vi "Transistor_Test.vi"() -> ()   [LabVIEW 2020]
panel:
  in  "?":T1(tab)
  in  "?":bool=TRUE
  out "Output Characteristics":cluster{dbl[], dbl[]}[](graph)
  in  "?":bool
  out "?":dbl(knob) scale=0.0..50.0
  out "Temperatur / C":dbl format="%#.2f"
  out "UC/Volt":dbl format="%#.2f"
  out "UB/Volt":dbl format="%#.2f"
  out "UCE/Volt":dbl format="%#.2f"
  out "UBE/Volt":dbl format="%#.2f"
  out "U Rc/Volt":dbl format="%#.2f"
  out "IC/mA":dbl format="%#.2f"
  out "IB/mA":dbl format="%#.2f"
  # "Project Name: Output Characteristics of Bipolar Transistor"
  # "Software : NI LabVIEW 2020\nVersion : 20.0 (32 bit)"
  # "Project Name: Output Characteristics of Bipolar Transistor"
  # "Current Monitoring display"
  # "Voltage Monitoring Display"
  # "Temperature Meter"
  # "Software : NI LabVIEW 2020\nVersion : 20.0 (32 bit)"
  # "Hochschule Bremen\n          Measurement and Instrumentation (MIN) \n                               Winter 2023/24      \nProject Name: Output characteristics of bipolar transistor\n      \nGuided By: \nProf. Dr. Friedrich Fleischmann\nDipl. Ing. Rene Ramson\n\nSubmitted by,\n1. MD JAHANGIR ALAM - 5300396\n2. EMDADUL HOQUE      - 5172827"
  # "Software : NI LabVIEW 2020\nVersion : 20.0 (32 bit)"
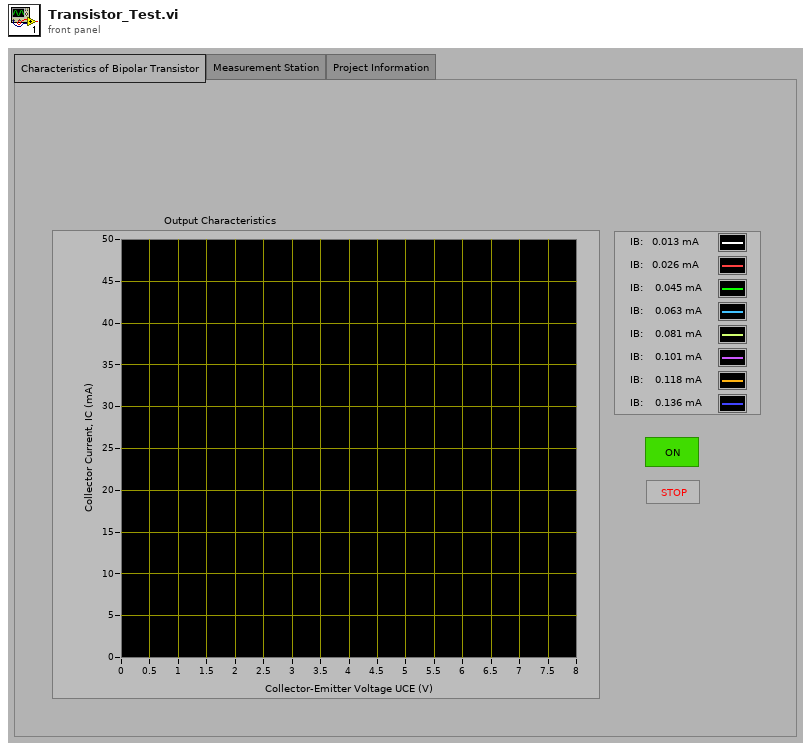
[diagram p1: front panel]
types:
  T1 = enum32{"Characteristics of Bipolar Transistor", "Measurement Station", "Project Information"}
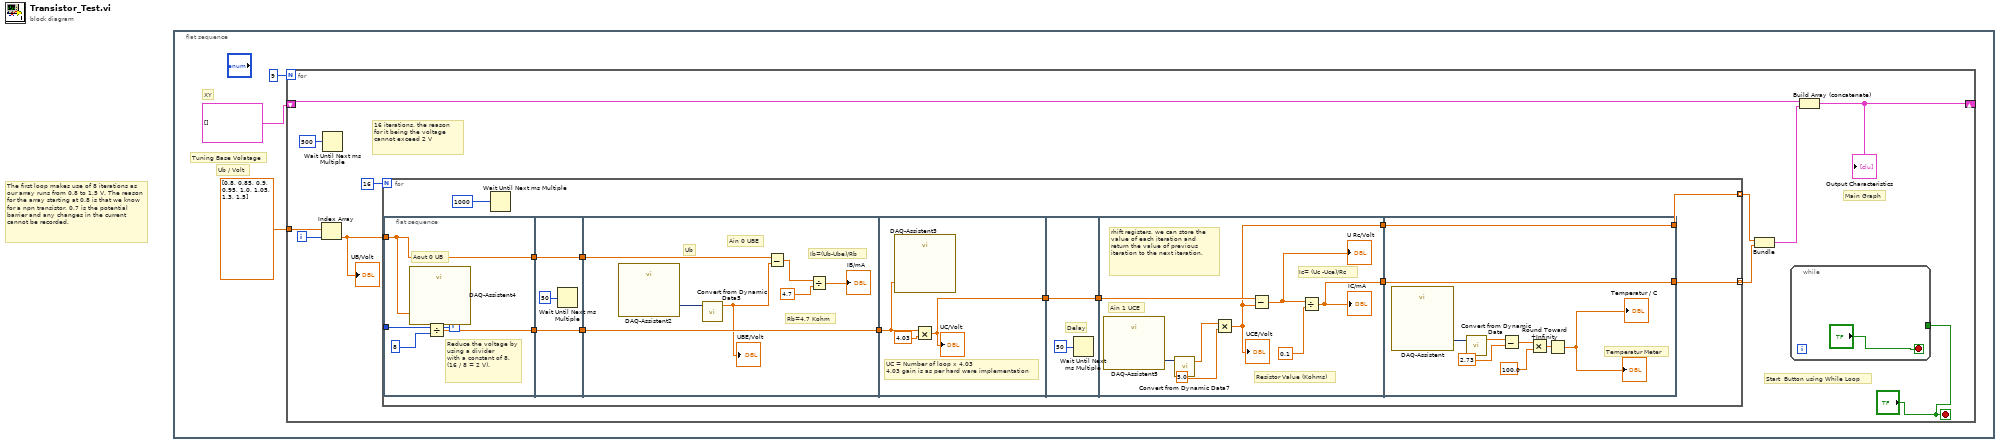
[diagram p0: block diagram]
diagram:
  # "The first loop makes use of 8 iterations as our array runs from 0.8 to 1.5 V. The reason for the array starting at 0.8 is that we know for a npn transistor, 0.7 is the potential barrier and any changes in the current cannot be recorded."
  n1 = flat-sequence {
    frame #0 {
      # "Tuning Base Volatage"
      # "XY"
      # "Ub / Volt"
      n2 = for {
        N: 9 -> [_]
        tunnel: dbl[] [0.8, 0.85, 0.9, 0.95, 1.0, 1.05, 1.3, 1.5] -> [w14]
        shift-right: [w7] -> _
        shift-left: cluster{dbl[], dbl[]}[] [] -> [w5]
        i -> [w12]
        stop <- "?" stop-if-true
        # "16 iterations, the reason for it being the voltage cannot exceed 2 V"
        # "Start  Button using While Loop"
        # "Main Graph"
        n3 = Index Array(array=w14, index=w12) -> (element=w10:dbl)
        "UB/Volt" <- w10
        n4 = Wait Until Next ms Multiple(millisecond multiple=u32 500) -> ()  [unwired: 1 out]
        n5 = for {
          N: 16 -> [_]
          tunnel: [w16] -> w9 mode=indexing
          tunnel: [w29] -> w8 mode=indexing
          tunnel: w10 -> [w25]
          i -> [w21]
          n6 = flat-sequence {
            tunnel: w21 -> [w33]
            tunnel: [w30] -> w27
            tunnel: w25 -> [w31]
            tunnel: [w31] -> w26
            tunnel: [w36] -> w20
            tunnel: [w35] -> w19
            tunnel: w27 -> [w36]
            tunnel: w26 -> [w35]
            tunnel: [w40] -> w28
            tunnel: w19 -> [w39]
            tunnel: w20 -> [w40]
            tunnel: [w44] -> w23
            tunnel: w28 -> [w45]
            tunnel: w23 -> [w48]
            tunnel: [w48] -> w22
            tunnel: w22 -> [w52]
            tunnel: [w51] -> w18
            tunnel: [w49] -> w17
            tunnel: [w64] -> w16
            tunnel: [w65] -> w29
            tunnel: w18 -> [w65]
            tunnel: w17 -> [w64]
            frame #0 {
              # "Reduce the voltage by using a divider\nwith a constant of 8. (16 / 8 = 2 V)."
              # "Aout 0 UB"
              n7 = call "DAQ-Assistent4"("data"=w31) -> ()  [unwired: 17 in, 2 out]
              n8 = Divide(x=w33, y=8) -> (x/y=w30:dbl)
            }
            frame #1 {
              n9 = Wait Until Next ms Multiple(millisecond multiple=u32 50) -> ()  [unwired: 1 out]
            }
            frame #2 {
              # "Rb=4.7 Kohm"
              # "Ib=(Ub-Ube)/Rb"
              # "Ub"
              # "Ain 0 UBE"
              n10 = call "DAQ-Assistent2"() -> ("data"=w38:dynamicdata)  [unwired: 17 in, 2 out]
              n11 = call "Convert from Dynamic Data5"("Dynamic Data Type"=w38) -> ("Scalar"=w37:dbl)  [unwired: 1 in, 2 out]
              "UBE/Volt" <- w37
              n12 = Subtract(x=w39, y=w37) -> (x-y=w43:dbl)
              n13 = Divide(x=w43, y=4.7) -> (x/y=→"IB/mA":dbl)
            }
            frame #3 {
              # "UC = Number of loop x 4,03\n4.03 gain is as per hard ware implementation"
              n14 = call "DAQ-Assistent3"("data"=w45) -> ()  [unwired: 17 in, 2 out]
              n15 = Multiply(x=w45, y=4.03) -> (x*y=w44:dbl)
              "UC/Volt" <- w44
            }
            frame #4 {
              # "Delay"
              n16 = Wait Until Next ms Multiple(millisecond multiple=u32 50) -> ()  [unwired: 1 out]
            }
            frame #5 {
              # "rhift registers, we can store the value of each iteration and\nreturn the value of previous iteration to the next iteration."
              # "Ic= (Uc -Uce)/Rc"
              # "Resistor Value (Kohms)"
              # "Ain 1 UCE"
              n17 = call "DAQ-Assistent5"() -> ("data"=w56:dynamicdata)  [unwired: 17 in, 2 out]
              n18 = call "Convert from Dynamic Data7"("Dynamic Data Type"=w56) -> ("Scalar"=w55:dbl)  [unwired: 1 in, 2 out]
              n19 = Multiply(x=w55, y=5.0) -> (x*y=w49:dbl)
              "UCE/Volt" <- w49
              n20 = Subtract(x=w52, y=w49) -> (x-y=w50:dbl)
              "U Rc/Volt" <- w50
              n21 = Divide(x=w50, y=0.1) -> (x/y=w51:dbl)
              "IC/mA" <- w51
            }
            frame #6 {
              # "Temperatur Meter"
              n22 = call "DAQ-Assistent"() -> ("data"=w63:dynamicdata)  [unwired: 17 in, 2 out]
              n23 = call "Convert from Dynamic Data"("Dynamic Data Type"=w63) -> ("Scalar"=w62:dbl)  [unwired: 1 in, 2 out]
              n24 = Subtract(x=w62, y=2.73) -> (x-y=w60:dbl)
              n25 = Multiply(x=w60, y=100.0) -> (x*y=w58:dbl)
              n26 = Round Toward +Infinity(x=w58) -> (ceil(x): smallest int >= x=→"Temperatur / C" →"?":dbl)
            }
          }
          n27 = Wait Until Next ms Multiple(millisecond multiple=u32 1000) -> ()  [unwired: 1 out]
        }
        n28 = Bundle(w9, w8) -> (w6:cluster{dbl[], dbl[]})  [unwired: 1 in]
        n29 = while {
          tunnel: "?" -> [_]
          stop <- "?" stop-if-true
        }
        n30 = Build Array (concatenate)(w5, w6) -> (w7:cluster{dbl[], dbl[]}[])
        "Output Characteristics" <- w7
      }
    }
  }
